vi "DataPointToPlot7.vi"(0 "Data ID in":i32, 1 "Cluster":cluster{"Time":u32, "Value":sgl}) -> ()   [LabVIEW 2013]
uses:
  GlobalNumPlotPoints.vi
  GlobalNumPlotChannels.vi
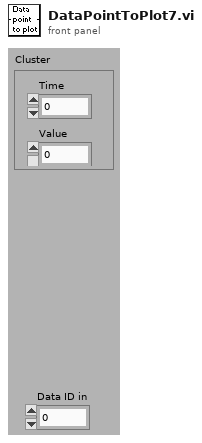
[diagram p1: front panel]
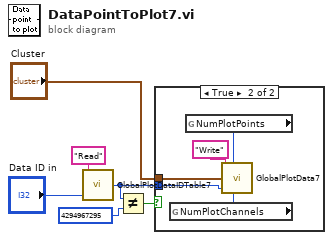
[diagram p0: block diagram]
diagram:
  n1 = call "GlobalPlotDataIDTable7.vi"("IO Data ID in"="Data ID in", "Function select"="Read") -> ("Plot channel out"=w3:u32)  [unwired: 2 in]
  n2 = Not Equal?(x=w3, y=u32 4294967295) -> (x != y?=w4:bool)
  n3 = case shown="True" w4 {
    tunnel: "Cluster" -> [_ w10]
    tunnel: w3 -> [_ w7]
    frame False {
    }
    frame True {
      n4 = global read "GlobalNumPlotChannels.vi" "NumPlotChannels"() -> (w8:i32)
      n5 = global read "GlobalNumPlotPoints.vi" "NumPlotPoints"() -> (w9:i32)
      n6 = call "GlobalPlotData7.vi"("Function select"="Write", "# Plot points"=w9, "IO data point in"=w10, "Data channel #"=w7, "# Data channels"=w8) -> ()  [unwired: 1 out]
    }
  }
